vi "OxITC503 _Config_ Control Sensor.vi"(2 "error in":errorcluster, 3 "Control Sensor":enum16{"Sensor 1", "Sensor 2", "Sensor 3"}(ring), 4 "VISA session":refnum<visa-resource-name>) -> (0 "error out (no error)":errorcluster, 1 "VISA session":refnum<visa-resource-name>)   [LabVIEW 2013]
doc: "Defines de sensor to be used for automatic control."
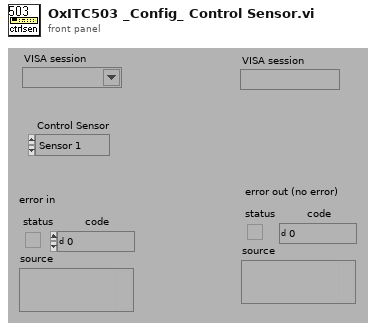
[diagram p1: front panel]
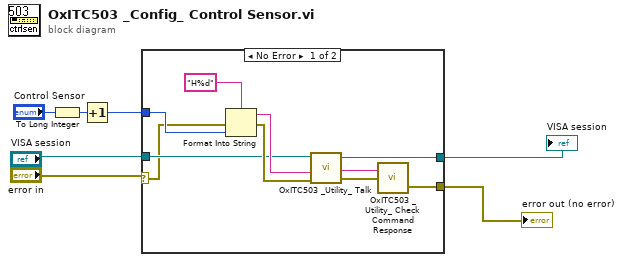
[diagram p0: block diagram]
diagram:
  n1 = To Long Integer(number="Control Sensor") -> (32bit integer=w2:i32)
  n2 = Increment(x=w2) -> (x+1=w3:i32)
  n3 = case shown="No Error" "error in" {
    selector: "error in" -> [w8 w18]
    tunnel: [w14 w19] -> w7
    tunnel: "VISA session" -> [w13 w19]
    tunnel: [w10 w18] -> w4
    tunnel: w3 -> [w9 _]
    frame No Error {
      n4 = Format Into String(format string="H%d" ("Format String"), error in=w8, w9) -> (resulting string=w16:string, error out=w17:errorcluster)  [unwired: 1 in]
      n5 = call "OxITC503 _Utility_ Talk.vi"("VISA session"=w13, "Command"=w16, "error in (no error)"=w17) -> ("VISA session"=w14:refnum<visa-resource-name>, "read buffer"=w11:string, "error out (no error)"=w12:errorcluster)  [unwired: 2 in]
      n6 = call "OxITC503 _Utility_ Check Command Response.vi"("error in"=w12, "read buffer"=w11) -> ("error out (no error)"=w10:errorcluster)  [unwired: 1 out]
    }
    frame Error {
    }
  }
  "error out (no error)" <- w4
  "VISA session" <- w7
